vi "EXPT_DILUTE.vi"(4 "Mixing pump frequency":dbl, 6 "Pump cycles for dilution":i32=40, 7 "Rings to load":T1, 8 "error in (no error)":errorcluster, 9 "ITT":dbl, 10 "Buffer":dbl, 11 ".NET Refnum in":refnum<k24>) -> (0 "error out":errorcluster, 3 ".NET Refnum out":refnum<k24>)   [LabVIEW 2018]
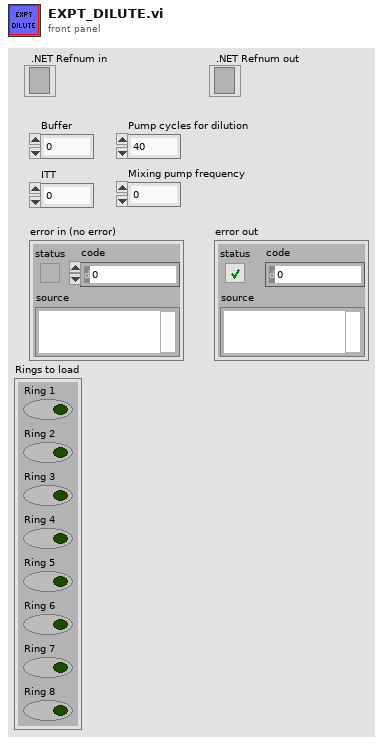
[diagram p1: front panel]
types:
  T1 = cluster{"Ring 1":bool, "Ring 2":bool, "Ring 3":bool, "Ring 4":bool, "Ring 5":bool, "Ring 6":bool, "Ring 7":bool, "Ring 8":bool}
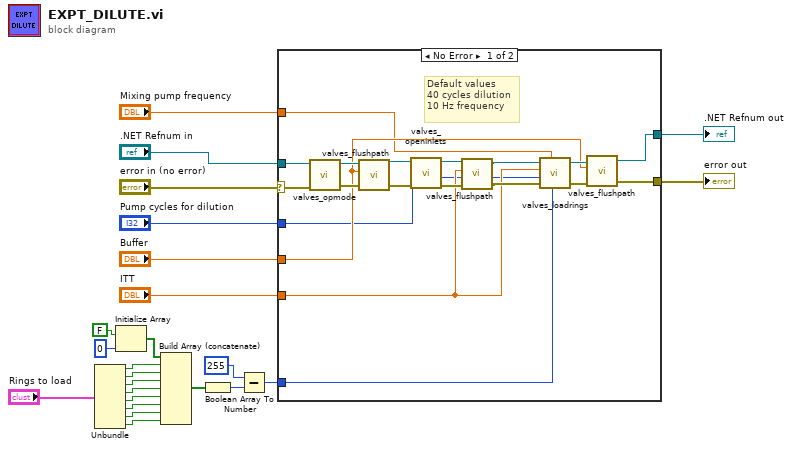
[diagram p0: block diagram]
diagram:
  n1 = Unbundle("Rings to load") -> ("Ring 1"=w3:bool, "Ring 2"=w4:bool, "Ring 3"=w5:bool, "Ring 4"=w6:bool, "Ring 5"=w7:bool, "Ring 6"=w8:bool, "Ring 7"=w9:bool, "Ring 8"=w10:bool)
  n2 = Initialize Array(FALSE, 0 ("dimension size")) -> (w19:bool[])
  n3 = Build Array (concatenate)(w19, w3, w4, w5, w6, w7, w8, w9, w10) -> (w18:bool[])
  n4 = Boolean Array To Number(Boolean array=w18) -> (number=w16:u32)
  n5 = Subtract(x=u32 255, y=w16) -> (x-y=w21:u32)
  n6 = case shown="No Error" "error in (no error)" {
    selector: "error in (no error)" -> [w36 w44]
    tunnel: "ITT" -> [w27 _]
    tunnel: "Buffer" -> [w37 _]
    tunnel: w21 -> [w35 _]
    tunnel: [w34 w44] -> w22
    tunnel: ".NET Refnum in" -> [w33 w45]
    tunnel: [w32 w45] -> w24
    tunnel: "Pump cycles for dilution" -> [w26 _]
    tunnel: "Mixing pump frequency" -> [w25 _]
    frame No Error {
      # "Default values\n40 cycles dilution\n10 Hz frequency"
      n7 = call "valves_opmode.vi"("COM4 in"=w33, "error in"=w36) -> ("COM4 out"=w43:refnum<k24>, "error out"=w42:errorcluster)  [unwired: 5 in]
      n8 = call "valves_flushpath.vi"("COM4 in"=w43, "Input solution"=w37, "error in"=w42) -> ("COM4 out"=w40:refnum<k24>, "error out"=w41:errorcluster)  [unwired: 4 in]
      n9 = call "valves_openinlets.vi"("error in"=w41, "COM4 in"=w40) -> ("error out"=w29:errorcluster, "COM4 out"=w31:refnum<k24>)  [unwired: 4 in]
      n10 = call "valves_flushpath.vi"("COM4 in"=w31, "Input solution"=w27, "error in"=w29) -> ("COM4 out"=w30:refnum<k24>, "error out"=w28:errorcluster)  [unwired: 4 in]
      n11 = call "valves_loadrings.vi"("COM4 in"=w30, "Frequency"=w25, "Input solution"=w27, "Cycles"=w26, "Rings to open"=w35, "error in"=w28) -> ("COM4 out"=w39:refnum<k24>, "error out"=w38:errorcluster)  [unwired: 1 in]
      n12 = call "valves_flushpath.vi"("COM4 in"=w39, "Input solution"=w37, "error in"=w38) -> ("COM4 out"=w32:refnum<k24>, "error out"=w34:errorcluster)  [unwired: 4 in]
    }
    frame Error {
    }
  }
  "error out" <- w22
  ".NET Refnum out" <- w24
